vi "Read Color.vi"(8 "error in (no error)":errorcluster, 11 "Flags in":refnum<class "Flags.lvclass">) -> (0 "error out":errorcluster, 2 "Color":T1[](array[typedef]), 3 "Flags out":refnum<class "Flags.lvclass">)   [LabVIEW 2015, in "Flags.lvclass"]
uses:
  Flags.lvclass
  ColorEnum.ctl
  Flags.lvclass/Flags.ctl
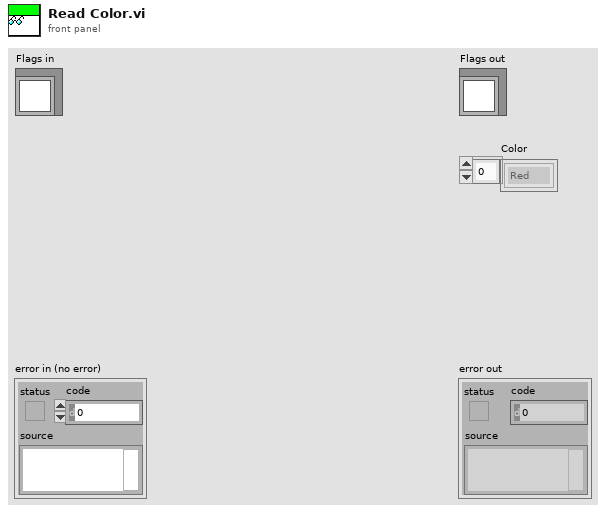
[diagram p1: front panel]
types:
  T1 = typedef "Flags.lvclass/ColorEnum.ctl" = enum8{"Red", "Blue", "Green", "Yellow"}
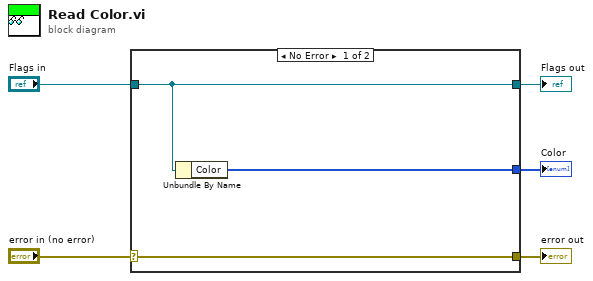
[diagram p0: block diagram]
diagram:
  n1 = case shown="No Error" "error in (no error)" {
    selector: "error in (no error)" -> [w8 w9]
    tunnel: [w8 w9] -> w4
    tunnel: [w7 w10] -> w2
    tunnel: "Flags in" -> [w7 w10]
    tunnel: [w6 _] -> w1
    frame No Error {
      n2 = Unbundle By Name(w7) -> ("Color"=w6:T1[])
    }
    frame Error {
    }
  }
  "error out" <- w4
  "Flags out" <- w2
  "Color" <- w1
